vi "2D Interpolation.vi"() -> ()   [LabVIEW 2023]
doc: "This example shows the operation of the 2D Interpolation VI. The interpolation parameters allow interactive changes to the interpolation method and the number of interpolation times."
uses:
  <vilib>/Math Plots/3D Math Plots/3D Surface/3D Surface XCtrl/3D Surface.xctl
  <vilib>/Math Plots/3D Math Plots/3D Plot/3D Plot/Typedef/Color Ramp Cluster.ctl
  <vilib>/Analysis/1siggen.llb/Ramp Pattern by Delta.vi
  <vilib>/gmath/interp.llb/Create Mesh Grid (2D) (x,y arrays).vi
  <vilib>/gmath/interp.llb/Interpolate 2D (1d X,Y).vi
  <vilib>/Math Plots/3D Math Plots/3D Surface/3D Surface Datatype/Public/Plot Helper (Matrix).vi
  <vilib>/gmath/NI_Gmath.lvlib
  <vilib>/Math Plots/3D Math Plots/3D Plot/3D Plot/3D Plot.lvclass
  <vilib>/Analysis/NI_AALBase.lvlib
  <vilib>/Math Plots/3D Math Plots/3D Surface/3D Surface Datatype/3D Surface Datatype.lvclass
panel:
  out "3D Surface":refnum<class "3D Plot Datatype.lvclass">[](xcontrol)
  in  "Color ramp style":T1(ring)=enum."Color spectrum"
  in  "Interpolated plot opacity":sgl(slide)=99.99 min=0 max=99.99 scale=0.0..100.0
  in  "Interpolation between n times":i32=2 min=1 max=4 step=1
  in  "Method":i32(ring)=3 items=["nearest", "bilinear", "bicubic", "bicubic spline"]
  in  "Stop":bool
  # "Overview: Demonstrates the operation of the Interpolate 2D VI.\nRequirements: LabVIEW Full Development System\nInstructions: \n1. Run the VI.\n2. Modify the Interpolation Settings and see how that affect the results of the graph and interpolated data on the 3D Surface.\n3. Click Stop to stop the VI."
  # "Interpolation Settings"
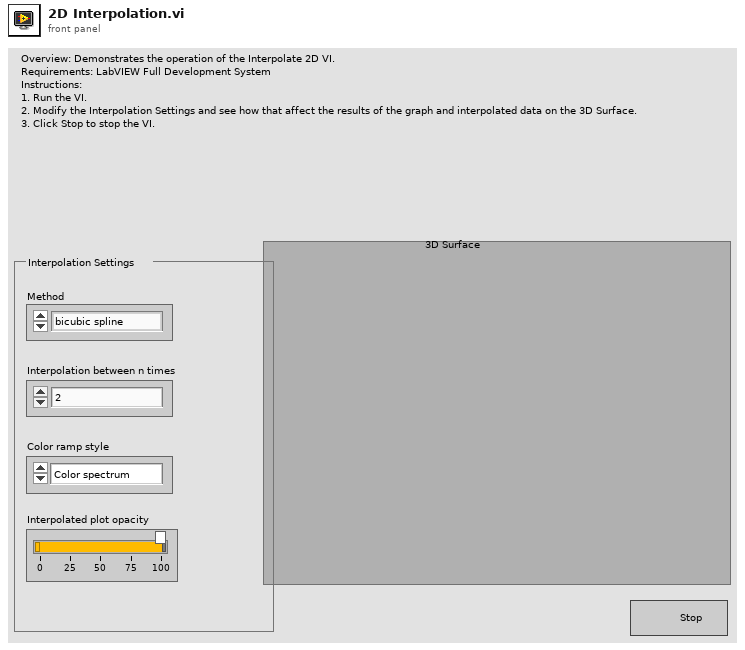
[diagram p1: front panel]
types:
  T1 = enum16{"None", "Shaded", "Color spectrum", "Grey scale", "Custom"}
  T2 = typedef "3D Plot.lvclass/Color Ramp Cluster.ctl" = cluster{"Color Ramp Style":enum16{"None", "Shaded", "Color spectrum", "Grey scale", "Custom"}, "Color Ramp Array":u32[], "Color Ramp Index":i32[], "Interpolate?":bool, "Logarithm?":bool}
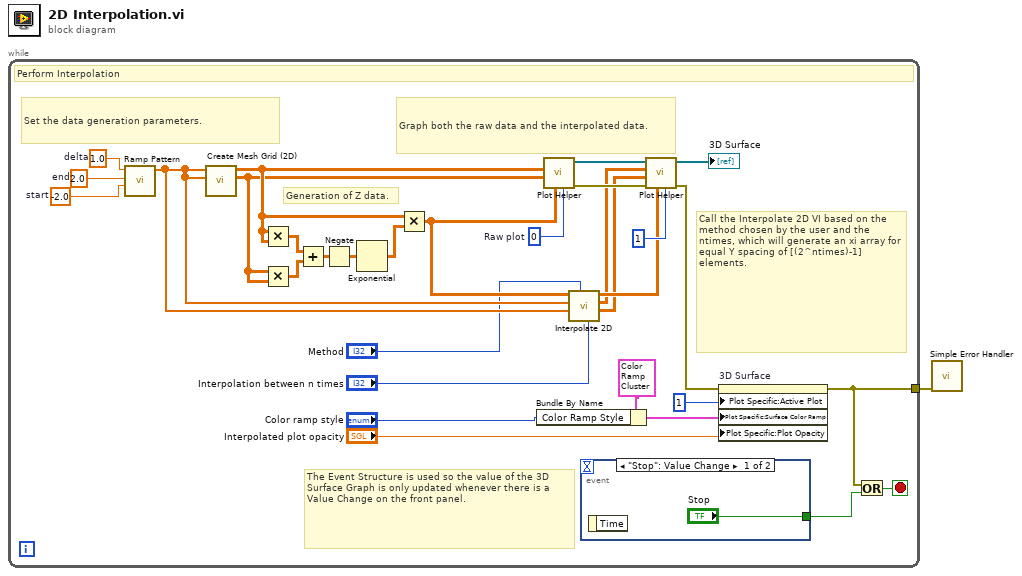
[diagram p0: block diagram]
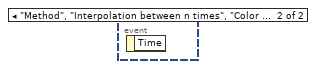
[diagram p2: hidden frame]
diagram:
  n1 = while {
    tunnel: [w4] -> w1
    stop <- w5 stop-if-true
    w17 = 0  # Raw plot
    w24 = 2.0  # end
    w25 = 1.0  # delta
    w23 = -2.0  # start
    # "The Event Structure is used so the value of the 3D Surface Graph is only updated whenever there is a Value Change on the front panel."
    # "Call the Interpolate 2D VI based on the method chosen by the user and the ntimes, which will generate an xi array for equal Y spacing of [(2^ntimes)-1] elements."
    # "Graph both the raw data and the interpolated data."
    # "Generation of Z data."
    # "Set the data generation parameters."
    # "Perform Interpolation"
    n2 = call-poly <vilib>:"Ramp Pattern.vi"("start"=w23, "end"=w24, "delta"=w25) -> ("Ramp Pattern"=w31:dbl[])  [unwired: 6 in, 2 out]
    n3 = call-poly <vilib>:"Create Mesh Grid (2D).vi"("y domain"=w31, "x domain"=w31) -> ("Y"=w19:dbl[][], "X"=w20:dbl[][])  [unwired: 7 in, 1 out]
    n4 = Multiply(x=w20, y=w20) -> (x*y=w26:dbl[][])
    n5 = Multiply(x=w19, y=w19) -> (x*y=w28:dbl[][])
    n6 = Add(x=w26, y=w28) -> (x+y=w29:dbl[][])
    n7 = Negate(x=w29) -> (-x=w27:dbl[][])
    n8 = Exponential(1:w27) -> (0:w30:dbl[][])
    n9 = Multiply(x=w20, y=w30) -> (x*y=w21:dbl[][])
    n10 = Bundle By Name(cluster=T2 {"Color Ramp Style"=enum."None", "Color Ramp Array"=[16711934, 393471, 57855, 4390754, 16449346, 16744722, 16711680], "Color Ramp Index"=[45, 91, 133, 175, 219, 255], "Interpolate?"=FALSE, "Logarithm?"=FALSE} ("Plot Specific:Surface:Surface Color Ramp"), "Color Ramp Style"="Color ramp style") -> (w9:T2)
    n11 = call-poly <vilib>:"Plot Helper.vi"("Plot ID"=w17, "z matrix"=w21, "y matrix"=w19, "x matrix"=w20) -> ("error out"=w15:errorcluster, "3D Plot lvclass Array out"=w18:refnum<class "3D Plot Datatype.lvclass">[])  [unwired: 2 in, 4 out]
    n12 = call-poly <vilib>:"Interpolate 2D.vi"("ntimes"="Interpolation between n times", "method"="Method", "Y"=w31, "X"=w31, "Z"=w21) -> ("yi used"=w12:dbl[][], "xi used"=w13:dbl[][], "zi"=w14:dbl[][])  [unwired: 3 in, 1 out]
    n13 = event shown="[0] \"Stop\": Value Change" {
      selector: _ -> [_ _]
      dyn-events: _ -> [_ _]
      timeout: _ -> [_ _]
      tunnel: ["Stop" _] -> w2
      event "Stop": Value Change {
        n14 = event-data() -> ()  [unwired: 1 in, 1 out]
      }
      event "Method", "Interpolation between n times", "Color ramp style", "Interpolated plot opacity": Value Change {
        n15 = event-data() -> ()  [unwired: 1 in, 1 out]
      }
    }
    n16 = call-poly <vilib>:"Plot Helper.vi"("Plot ID"=1, "z matrix"=w14, "error in (no error)"=w15, "y matrix"=w12, "x matrix"=w13, "3D Plot lvclass Array in"=w18) -> ("error out"=w6:errorcluster, "3D Plot lvclass Array out"=→"3D Surface":refnum<class "3D Plot Datatype.lvclass">[])  [unwired: 4 out]
    n17 = property on="3D Surface" class="3D Surface (strict)"(error in=w6, "Plot Specific:Active Plot"=1, "Plot Specific:Surface Color Ramp"=w9, "Plot Specific:Plot Opacity"="Interpolated plot opacity") -> (error out=w4:errorcluster)  [unwired: 1 in, 1 out]
    n18 = Or(x=w4, y=w2) -> (x .or. y?=w5:bool)
  }
  n19 = call <vilib>:"Simple Error Handler.vi"("error in (no error)"=w1) -> ()  [unwired: 4 in, 5 out]
